vi "Scan action.vi"(0 "Index":i32, 1 "Channels: AO":T1={"AO amp (V)"=[0.002, 0.002, 0.002, 0.002, 0.002, 0.002, 0.002, 0.002], "AO DC (V)"=[0.0, 0.0, 0.0, 0.0, 0.0, 0.0, 0.0, 0.0], "AO f (Hz)"=[15.1, 15.11, 15.12, 15.13, 15.14, 15.15, 15.16, 15.17], "AO phi (deg)"=[0.0, 10.0, 20.0, 30.0, 40.0, 50.0, 60.0, 70.0], "function"=[enum."Sine Wave", enum."Sine Wave", enum."Sine Wave", enum."Sine Wave", enum."Sine Wave", enum."Sine Wave", enum."Sine Wave", enum."Sine Wave"]} {"AO DC (V)" format="%#_6p"; "AO amp (V)" format="%#_6p"}, 2 "Scan control":T3=enum."Vsg1", 3 "Scan Parameters":T2={"DAQ Channel"=2, "Label"="\nscaledVsg1=", "Start"=0.14, "End"=-0.060000000000000005, "Step"=-0.060000000000000005, "B sweep rate"=-0.060000000000000005} {"B sweep rate" format="%.2f"; "Step" format="%#_6p"; "End" format="%#_6p"; "Start" format="%#_6p"}, 4 "Comments":string) -> (5 "Comments out":string, 6 "Channels: AO":T1={"AO amp (V)"=[0.002, 0.002, 0.002, 0.002, 0.002, 0.002, 0.002, 0.002], "AO DC (V)"=[0.0, 0.0, 0.0, 0.0, 0.0, 0.0, 0.0, 0.0], "AO f (Hz)"=[15.1, 15.11, 15.12, 15.13, 15.14, 15.15, 15.16, 15.17], "AO phi (deg)"=[0.0, 10.0, 20.0, 30.0, 40.0, 50.0, 60.0, 70.0], "function"=[enum."Sine Wave", enum."Sine Wave", enum."Sine Wave", enum."Sine Wave", enum."Sine Wave", enum."Sine Wave", enum."Sine Wave", enum."Sine Wave"]} {"AO DC (V)" format="%#_6p"; "AO amp (V)" format="%#_6p"}, 7 "Stop?":bool)   [LabVIEW 2016]
uses:
  Typedefs/Enum - Action.ctl
  Typedefs/Cluster - ScanParamters.ctl
panel:
  in  "Physical Channel(s)":tag="Dev2/ao0"
  in  "VISA resource name":refnum<visa-resource-name>="GPIB0::24::INSTR"
  in  "Rate (K/min)":dbl=5.0
  # "0"
  # "1"
  # "2"
  # "3"
  # "4"
  # "5"
  # "6"
  # "7"
  # "0"
  # "1"
  # "2"
  # "3"
  # "4"
  # "5"
  # "6"
  # "7"
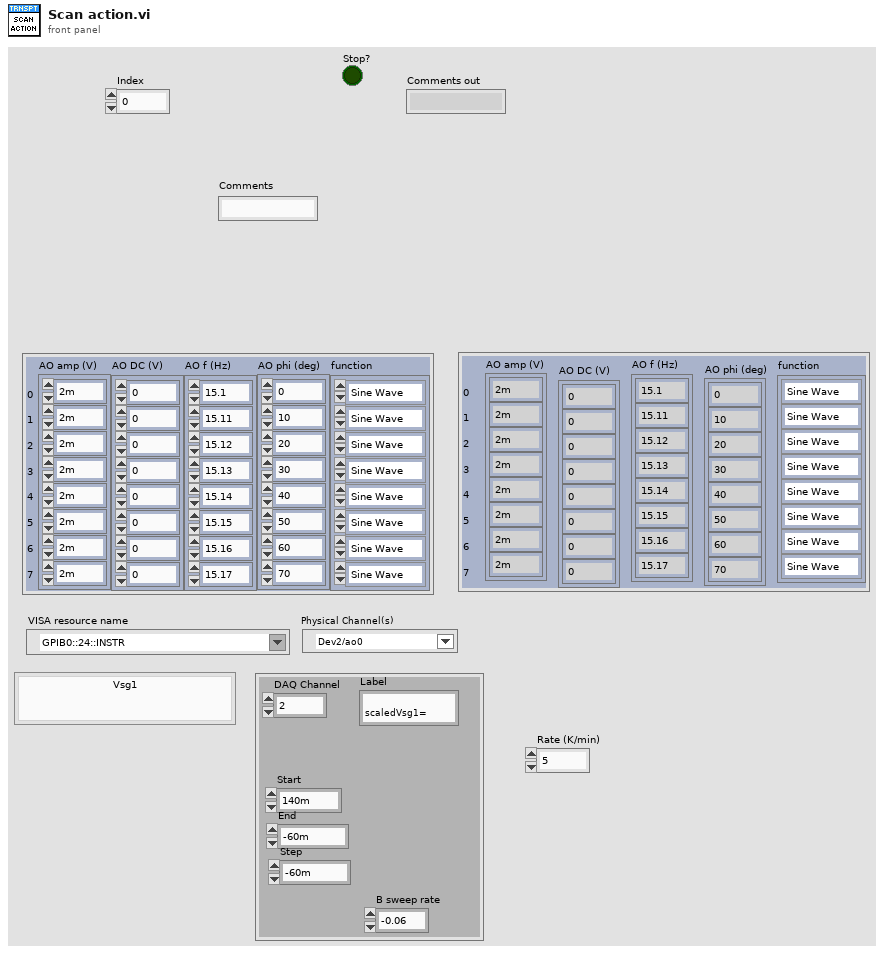
[diagram p1: front panel]
types:
  T1 = cluster{"AO amp (V)":dbl[], "AO DC (V)":dbl[], "AO f (Hz)":dbl[], "AO phi (deg)":dbl[], "function":enum16{"Sine Wave", "Triangle Wave", "Square Wave", "Sawtooth Wave"}[]}
  T2 = typedef "Cluster - ScanParamters.ctl" = cluster{"DAQ Channel":i32, "Label":string, "Start":dbl, "End":dbl, "Step":dbl, "B sweep rate":dbl}
  T3 = typedef "Enum - Action.ctl" = enum16{"OFF", "Vsg1", "Vsg2", "Vsgw", "Vbg", "Vamp", "Field", "Temp", "MW_freq", "MW_amplitude"}
  T4 = cluster{"Field (T)":dbl, "Sweep rate (T/min)":dbl}
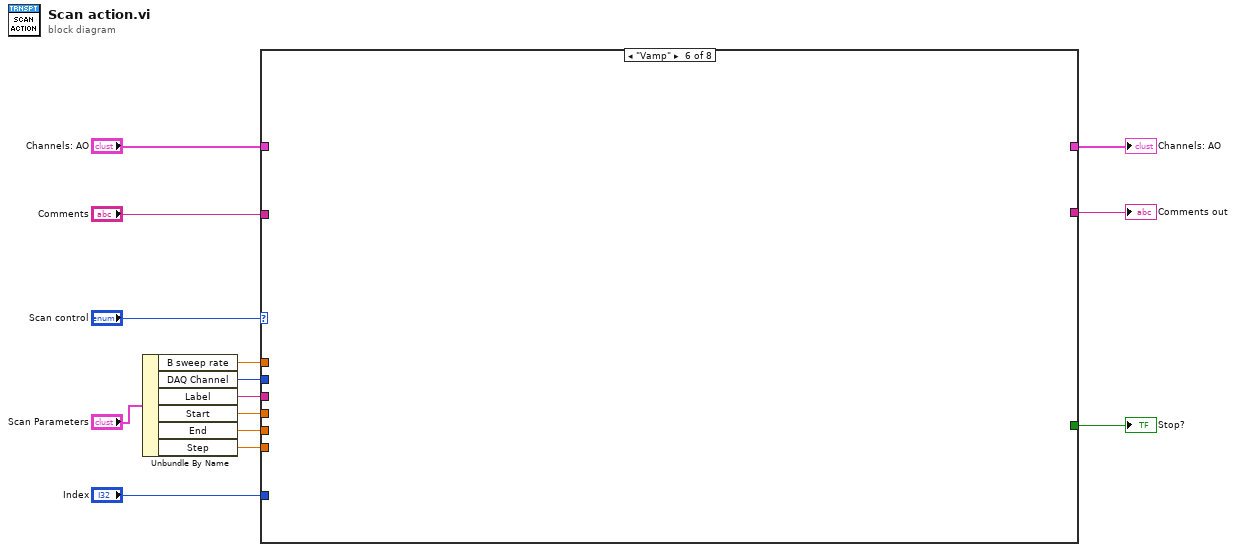
[diagram p0: block diagram]
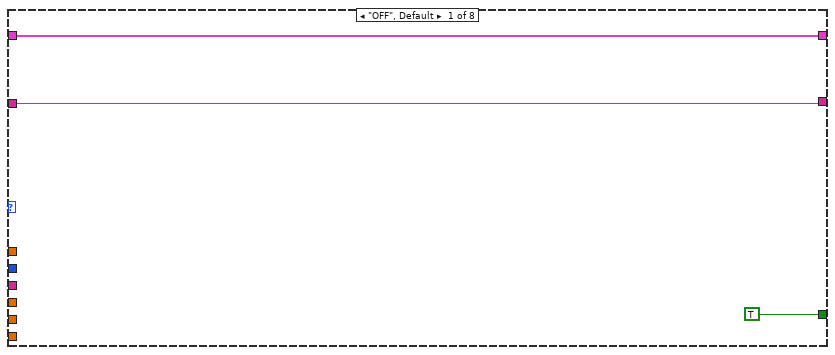
[diagram p2: hidden frame]
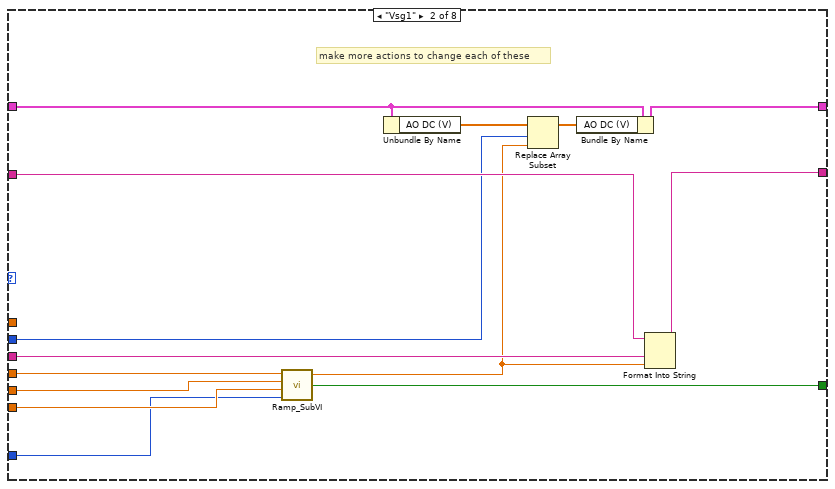
[diagram p3: hidden frame]
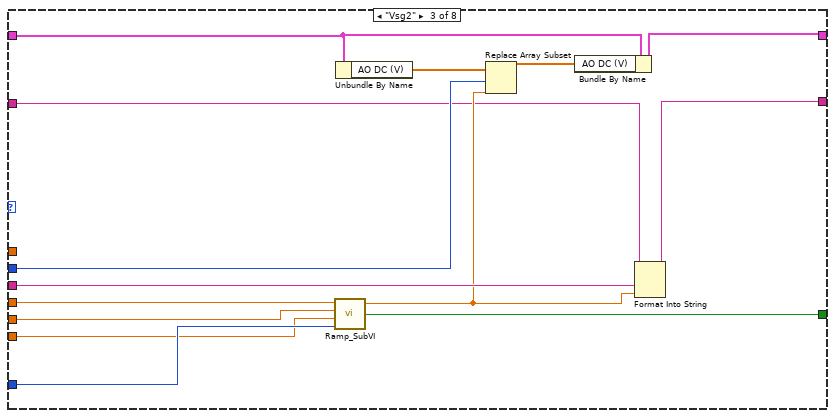
[diagram p4: hidden frame]
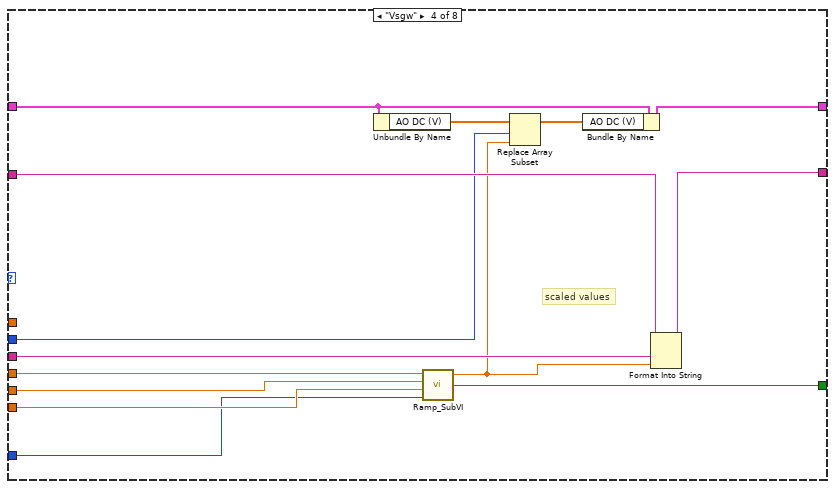
[diagram p5: hidden frame]
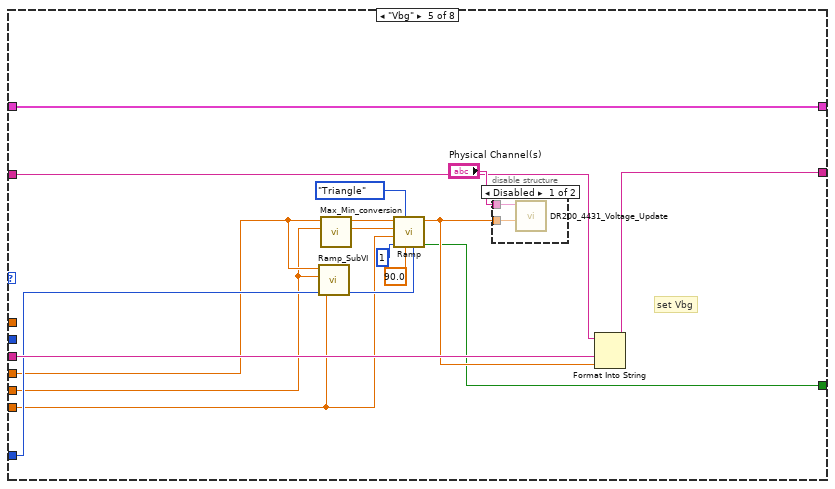
[diagram p6: hidden frame]
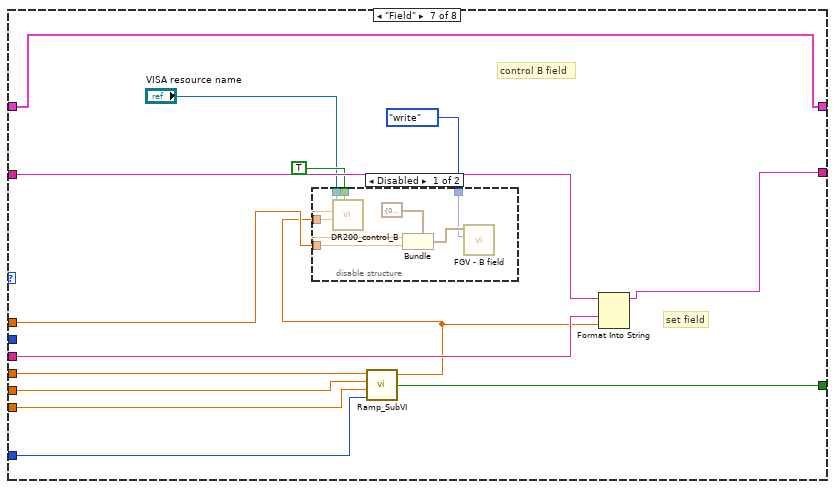
[diagram p8: hidden frame]
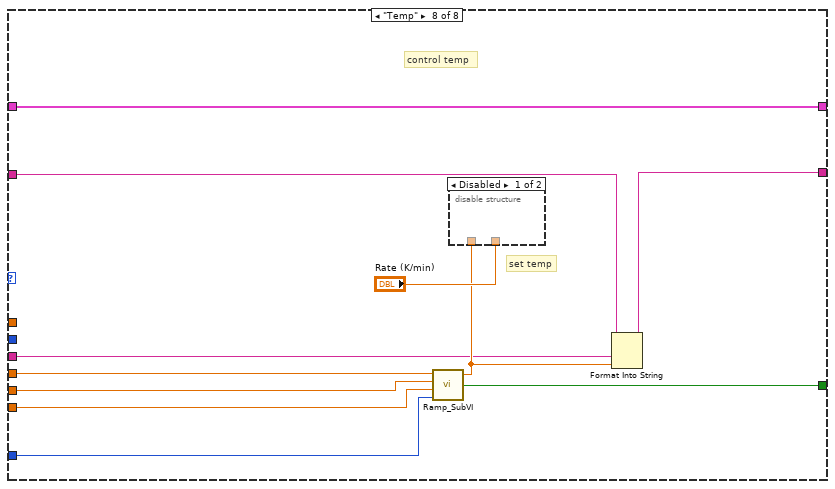
[diagram p10: hidden frame]
diagram:
  n1 = Unbundle By Name("Scan Parameters") -> ("B sweep rate"=w1:dbl, "DAQ Channel"=w9:i32, "Label"=w5:string, "Start"=w7:dbl, "End"=w6:dbl, "Step"=w8:dbl)
  n2 = case shown="\"Vamp\"" "Scan control" {
    tunnel: w9 -> [_ w19 w36 w46 _ _ _ _]
    tunnel: "Comments" -> [w17 w28 w33 w50 w63 _ w87 w100]
    tunnel: w5 -> [_ w27 w42 w55 w75 _ w86 w104]
    tunnel: "Index" -> [_ w21 w38 w48 w72 _ w80 w108]
    tunnel: w7 -> [_ w31 w45 w59 w67 _ w91 w102]
    tunnel: w6 -> [_ w20 w44 w58 w66 _ w90 w101]
    tunnel: w8 -> [_ w30 w37 w57 w65 _ w89 w109]
    tunnel: [TRUE ("Stop?") w29 w43 w56 w61 _ w88 w107] -> w3
    tunnel: [w17 w22 w32 w49 w60 _ w85 w99] -> w2
    tunnel: "Channels: AO" -> [w15 w18 w40 w52 w69 _ w84 w103]
    tunnel: [w15 w24 w34 w51 w69 _ w84 w103] -> w12
    tunnel: w1 -> [_ _ _ _ _ _ w79 _]
    frame "OFF", Default {
    }
    frame "Vsg1" {
      # "make more actions to change each of these"
      n3 = call <userlib>:"Ramp_SubVI.vi"("index"=w21, "step"=w30, "end"=w20, "start"=w31) -> ("Stop?"=w29:bool, "Numeric"=w23:dbl)  [unwired: 1 in]
      n4 = Unbundle By Name(w18) -> ("AO DC (V)"=w26:dbl[])
      n5 = Replace Array Subset(array=w26, new element=w23, index=w19) -> (w25:dbl[])
      n6 = Bundle By Name(cluster=w18, "AO DC (V)"=w25) -> (w24:T1)
      n7 = Format Into String(initial string=w28, w27, w23) -> (resulting string=w22:string)  [unwired: 2 in, 1 out]
    }
    frame "Vsg2" {
      n8 = call <userlib>:"Ramp_SubVI.vi"("index"=w38, "step"=w37, "end"=w44, "start"=w45) -> ("Stop?"=w43:bool, "Numeric"=w35:dbl)  [unwired: 1 in]
      n9 = Unbundle By Name(w40) -> ("AO DC (V)"=w41:dbl[])
      n10 = Replace Array Subset(array=w41, new element=w35, index=w36) -> (w39:dbl[])
      n11 = Bundle By Name(cluster=w40, "AO DC (V)"=w39) -> (w34:T1)
      n12 = Format Into String(initial string=w33, w42, w35) -> (resulting string=w32:string)  [unwired: 2 in, 1 out]
    }
    frame "Vsgw" {
      # "scaled values"
      n13 = Unbundle By Name(w52) -> ("AO DC (V)"=w54:dbl[])
      n14 = call <userlib>:"Ramp_SubVI.vi"("index"=w48, "step"=w57, "end"=w58, "start"=w59) -> ("Stop?"=w56:bool, "Numeric"=w47:dbl)  [unwired: 1 in]
      n15 = Replace Array Subset(array=w54, new element=w47, index=w46) -> (w53:dbl[])
      n16 = Bundle By Name(cluster=w52, "AO DC (V)"=w53) -> (w51:T1)
      n17 = Format Into String(initial string=w50, w55, w47) -> (resulting string=w49:string)  [unwired: 2 in, 1 out]
    }
    frame "Vbg" {
      # "set Vbg"
      n18 = call <userlib>:"Ramp_SubVI.vi"("index"=w72, "step"=w65, "end"=w66, "start"=w67) -> ()  [unwired: 1 in, 2 out]
      n19 = call <userlib>:"Max_Min_conversion.vi"("Min"=w66, "Max"=w67) -> ("offset"=w73:dbl, "Amplitude"=w74:dbl)  [unwired: 8 in]
      n20 = call <userlib>:"Ramp.vi"("i"=w72, "phase"=90.0, "function (ramp)"=enum16{"Ramp", "Triangle", "Sine"}."Triangle", "cycles (1,2,...)"=1, "step size"=w65, "offset"=w73, "amplitude"=w74) -> ("stop?"=w61:bool, "element"=w62:dbl)  [unwired: 2 in, 1 out]
      n21 = disable-structure shown="Disabled" {
        disable-tunnel: "Physical Channel(s)" -> [w77 _]
        disable-tunnel: w62 -> [w76 _]
        frame Disabled {
          n22 = call "DR200_4431_Voltage_Update.vi"("Amplified output"=w76, "Physical Channel(s)"=w77) -> ()  [unwired: 10 in]
        }
        frame Enabled {
        }
      }
      n23 = Format Into String(initial string=w63, w75, w62) -> (resulting string=w60:string)  [unwired: 2 in, 1 out]
    }
    frame "Vamp" {
    }
    frame "Field" {
      # "control B field"
      # "set field"
      n24 = call <userlib>:"Ramp_SubVI.vi"("index"=w80, "step"=w89, "end"=w90, "start"=w91) -> ("Stop?"=w88:bool, "Numeric"=w78:dbl)  [unwired: 1 in]
      n25 = disable-structure shown="Disabled" {
        disable-tunnel: TRUE ("wait for  B?") -> [w98 _]
        disable-tunnel: "VISA resource name" -> [w97 _]
        disable-tunnel: enum16{"write", "read"}."write" ("Function") -> [w94 _]
        disable-tunnel: w79 -> [w93 _]
        disable-tunnel: w78 -> [w92 _]
        frame Disabled {
          n26 = call "DR200_control_B.vi"("wait for  B?"=w98, "set B (T)"=w92, "sweep rate (T/min)"=w93, "VISA resource name"=w97) -> ()  [unwired: 6 in, 2 out]
          n27 = Bundle(cluster=T4 {"Field (T)"=0.0, "Sweep rate (T/min)"=0.0} ("output cluster"), "Field (T)"=w92, "Sweep rate (T/min)"=w93) -> (w95:T4)
          n28 = call "FGV - B field.vi"("Function"=w94, "output cluster"=w95) -> ()  [unwired: 4 in, 2 out]
        }
        frame Enabled {
        }
      }
      n29 = Format Into String(initial string=w87, w86, w78) -> (resulting string=w85:string)  [unwired: 2 in, 1 out]
    }
    frame "Temp" {
      # "control temp"
      # "set temp"
      n30 = call <userlib>:"Ramp_SubVI.vi"("index"=w108, "step"=w109, "end"=w101, "start"=w102) -> ("Stop?"=w107:bool, "Numeric"=w105:dbl)  [unwired: 1 in]
      n31 = disable-structure shown="Disabled" {
        disable-tunnel: "Rate (K/min)" -> [_ _]
        disable-tunnel: w105 -> [_ _]
        frame Disabled {
        }
        frame Enabled {
        }
      }
      n32 = Format Into String(initial string=w100, w104, w105) -> (resulting string=w99:string)  [unwired: 2 in, 1 out]
    }
  }
  "Comments out" <- w2
  "Stop?" <- w3
  "Channels: AO" <- w12
